vi "Add_Second_To_Timestamp.vi"(8 "Status/Errors in":refnum<vi>, 9 "Add/Subtract":T3, 10 "Time stamp":T2, 11 "Master?":T1) -> (0 "Status/Errors out":refnum<vi>, 2 "Time stamp out":T2, 3 "Timestamp OK?":bool)   [LabVIEW 2010]
uses:
  Controls/GPS_Timestamp.ctl
  Controls/Add_Subtract.ctl
  Controls/Master.ctl
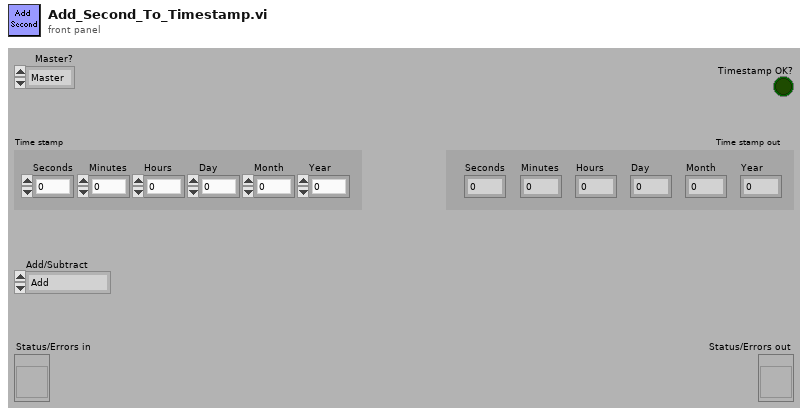
[diagram p1: front panel]
types:
  T1 = typedef "Master.ctl" = enum16{"Master", "Slave", "General"}
  T2 = typedef "GPS_Timestamp.ctl" = cluster{"Seconds":u8, "Minutes":u8, "Hours":u8, "Day":u8, "Month":u8, "Year":u16}
  T3 = typedef "Add_Subtract.ctl" = enum16{"Add", "Subtract"}
  T4 = cluster{"second":i32, "minute":i32, "hour":i32, "day of month":i32, "month":i32, "year":i32, "day of week":i32, "day of year":i32, "is DST":i32}
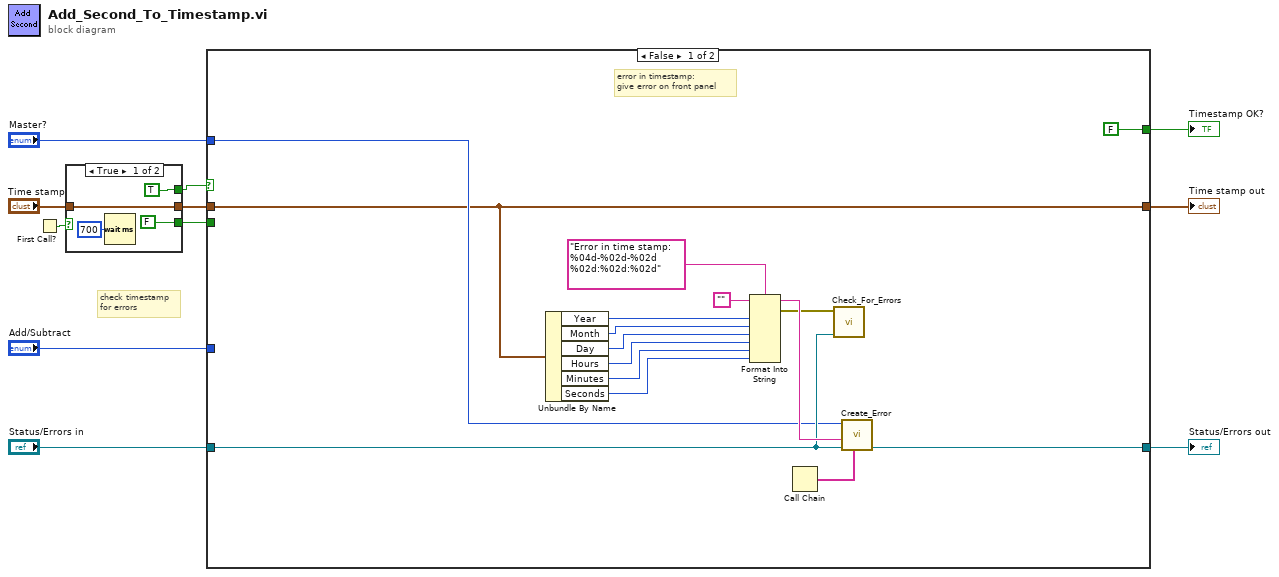
[diagram p0: block diagram]
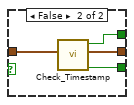
[diagram p2: hidden frame]
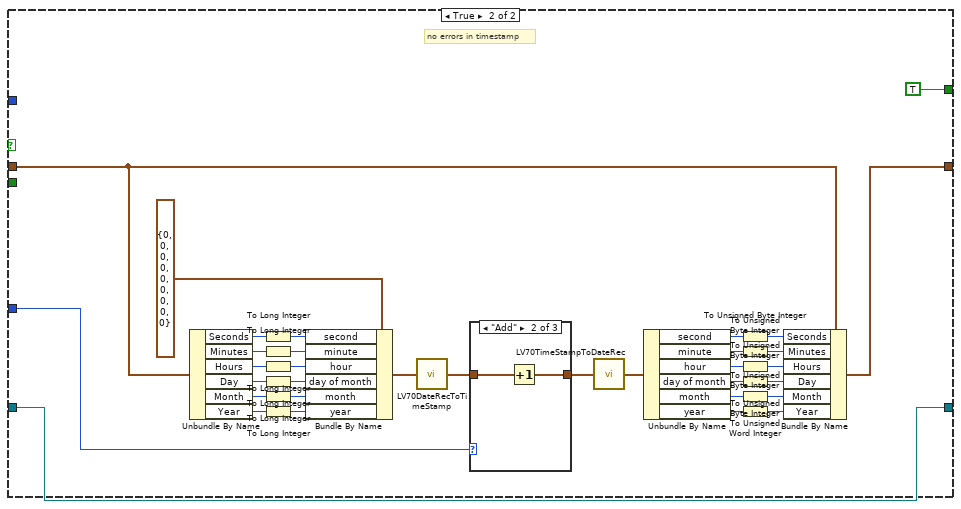
[diagram p3: hidden frame]
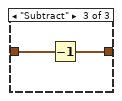
[diagram p5: hidden frame]
diagram:
  # "check timestamp\nfor errors"
  n1 = First Call?() -> (First Call?: T/F=w1:bool)
  n2 = case shown="True" w1 {
    tunnel: "Time stamp" -> [w13 w19]
    tunnel: [FALSE ("Leap year?") w18] -> w8
    tunnel: [TRUE ("Result") w17] -> w7
    tunnel: [w13 w16] -> w3
    frame True {
      n3 = Wait (ms)(milliseconds to wait=u32 700) -> ()  [unwired: 1 out]
    }
    frame False {
      n4 = call "Check_Timestamp.vi"("Time stamp in"=w19) -> ("Leap year?"=w18:bool, "Time stamp out"=w16:T2, "Result"=w17:bool)  [unwired: 8 out]
    }
  }
  n5 = case shown="False" w7 {
    tunnel: [w21 w38] -> w11
    tunnel: "Add/Subtract" -> [_ w55]
    tunnel: w3 -> [w21 w39]
    tunnel: w8 -> [_ _]
    tunnel: "Status/Errors in" -> [w24 w37]
    tunnel: [w23 w37] -> w5
    tunnel: "Master?" -> [w22 _]
    tunnel: [FALSE TRUE] -> w2
    frame False {
      # "error in timestamp:\ngive error on front panel"
      n6 = Unbundle By Name(w21) -> ("Year"=w32:u16, "Month"=w31:u8, "Day"=w30:u8, "Hours"=w29:u8, "Minutes"=w28:u8, "Seconds"=w27:u8)
      n7 = Format Into String(format string="Error in time stamp: %04d-%02d-%02d %02d:%02d:%02d", initial string="", w32, w31, w30, w29, w28, w27) -> (resulting string=w26:string, error out=w25:errorcluster)  [unwired: 1 in]
      n8 = Call Chain() -> (call chain=w35:string[])
      n9 = call "Check_For_Errors.vi"("Status/Errors in"=w24, "error in"=w25) -> ()  [unwired: 10 out]
      n10 = call "Create_Error.vi"("Call chain"=w35, "Status/Errors in"=w24, "HiSPARC error"=w26, "Master?"=w22) -> ("Status/Errors out"=w23:refnum<vi>)  [unwired: 2 in, 5 out]
    }
    frame True {
      # "no errors in timestamp"
      n11 = Unbundle By Name(w39) -> ("Seconds"=w68:u8, "Minutes"=w67:u8, "Hours"=w66:u8, "Day"=w65:u8, "Month"=w64:u8, "Year"=w63:u16)
      n12 = To Long Integer(number=w68) -> (32bit integer=w62:i32)
      n13 = To Long Integer(number=w67) -> (32bit integer=w61:i32)
      n14 = To Long Integer(number=w66) -> (32bit integer=w60:i32)
      n15 = To Long Integer(number=w65) -> (32bit integer=w59:i32)
      n16 = To Long Integer(number=w64) -> (32bit integer=w58:i32)
      n17 = To Long Integer(number=w63) -> (32bit integer=w57:i32)
      n18 = Bundle By Name(cluster=T4 {"second"=0, "minute"=0, "hour"=0, "day of month"=0, "month"=0, "year"=0, "day of week"=0, "day of year"=0, "is DST"=0} ("date time rec"), "second"=w62, "minute"=w61, "hour"=w60, "day of month"=w59, "month"=w58, "year"=w57) -> (w56:T4)
      n19 = call <vilib>:"LV70DateRecToTimeStamp.vi"("date time rec"=w56) -> ("Time Stamp"=w54:timestamp)
      n20 = case shown="\"Add\"" w55 {
        tunnel: w54 -> [w70 w72 w74]
        tunnel: [w70 w71 w73] -> w53
        frame Default {
        }
        frame "Add" {
          n21 = Increment(x=w72) -> (x+1=w71:timestamp)
        }
        frame "Subtract" {
          n22 = Decrement(x=w74) -> (x-1=w73:timestamp)
        }
      }
      n23 = call <vilib>:"LV70TimeStampToDateRec.vi"("time stamp"=w53) -> ("date time rec"=w40:T4)
      n24 = Unbundle By Name(w40) -> ("second"=w52:i32, "minute"=w51:i32, "hour"=w50:i32, "day of month"=w49:i32, "month"=w48:i32, "year"=w47:i32)
      n25 = To Unsigned Byte Integer(number=w52) -> (unsigned 8bit integer=w46:u8)
      n26 = To Unsigned Byte Integer(number=w51) -> (unsigned 8bit integer=w45:u8)
      n27 = To Unsigned Byte Integer(number=w50) -> (unsigned 8bit integer=w44:u8)
      n28 = To Unsigned Byte Integer(number=w49) -> (unsigned 8bit integer=w43:u8)
      n29 = To Unsigned Byte Integer(number=w48) -> (unsigned 8bit integer=w42:u8)
      n30 = To Unsigned Word Integer(number=w47) -> (unsigned 16bit integer=w41:u16)
      n31 = Bundle By Name(cluster=w39, "Seconds"=w46, "Minutes"=w45, "Hours"=w44, "Day"=w43, "Month"=w42, "Year"=w41) -> (w38:T2)
    }
  }
  "Time stamp out" <- w11
  "Status/Errors out" <- w5
  "Timestamp OK?" <- w2
